vi "Get Department.vi"(8 "error in (no error)":errorcluster, 11 "SOL User in":refnum<class "SOL User.lvclass">) -> (0 "error out":errorcluster, 2 "Department":string, 3 "SOL User out":refnum<class "SOL User.lvclass">)   [LabVIEW 2020, in "Summer of LabVIEW.lvlib" / "SOL User.lvclass"]
uses:
  SOL User.lvclass
  SOL User.lvclass/SOL User.ctl
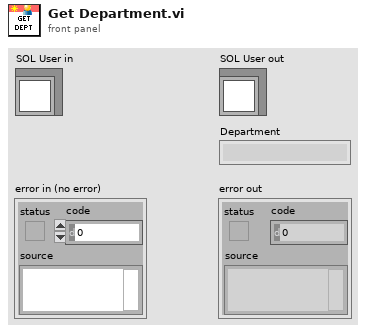
[diagram p1: front panel]
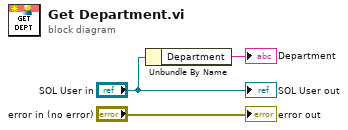
[diagram p0: block diagram]
diagram:
  n1 = Unbundle By Name("SOL User in") -> ("Department"=→"Department":string)
  "error out" <- "error in (no error)"
  "SOL User out" <- "SOL User in"
